vi "Run.vi"(8 "error in (no error)":errorcluster, 11 "S Parameter in":refnum<class "S Parameter.lvclass">) -> (0 "error out":errorcluster, 1 "Parameters":cluster{"Name":string, "Value":string}[](array[cluster]), 2 "Cancled":bool, 3 "S Parameter out":refnum<class "S Parameter.lvclass">)   [LabVIEW 2020, in "S Parameter.lvclass"]
doc: "This is the main test vi. It is here that the test is implemented."
uses:
  S Parameter.lvclass
  C:/Sandbox/Git_Sandbox/WiSpry Test Framework source code (LV20)/WiSpry Test Framework/Measurements/Measurement.lvclass
  Instruments/Vector Network Analyzer/Controls/Sparameter cluster.ctl
  Controls/Run States.ctl
  S Parameter.lvclass/S Parameter.ctl
  Instruments/Vector Network Analyzer/Vector Network Analyzer.lvclass/Vector Network Analyzer.ctl
  Instruments/Instrument.lvclass/Instrument.ctl
  Measurement.lvclass/Measurement.ctl
  XML Handler/XML Handler.lvclass/XML Handler.ctl
  Instruments/Power Supply/Power Supply.lvclass/Power Supply.ctl
  Devices/Controls/Change setting mode enum.ctl
  XML Handler/Controls/Result Cluster.ctl
  Instruments/Vector Network Analyzer/Vector Network Analyzer.lvclass
  C:/Sandbox/Git_Sandbox/WiSpry Test Framework source code (LV20)/WiSpry Test Framework/Instruments/Instrument.lvclass
  Support VI/Update parameters (array).vi
  Measurement.lvclass
  Devices/Device.lvclass
  Instruments/Power Supply/Power Supply.lvclass
  XML Handler/XML Handler.lvclass
  Devices/PIC-device/PIC-Device.lvclass
  Instruments/Digital Multimeter/Digital Multimeter.lvclass
  Instruments/Instrument.lvclass
  <vilib>/addons/HF Network Analysis/NI_HFNetworkAnalysis.lvlib
panel:
  out "S parameters":T1[](array[typedef])
  out "s-para plot error":errorcluster
  in  "S-par":u16(ring)
  in  "Format":u16(ring) items=["Ampl (dB)", "Ampl (mag)", "Phase (deg)", "Phase (rad)", "Re", "Im"]
  out "S-parameter Graph":T2(graph)
  out "Device Parameters":string
  out "Progress":u8(slide) scale=0.0..100.0
  in  "Cancel Button":bool
  out "Estimated finish time":timestamp format="%<%X>T"
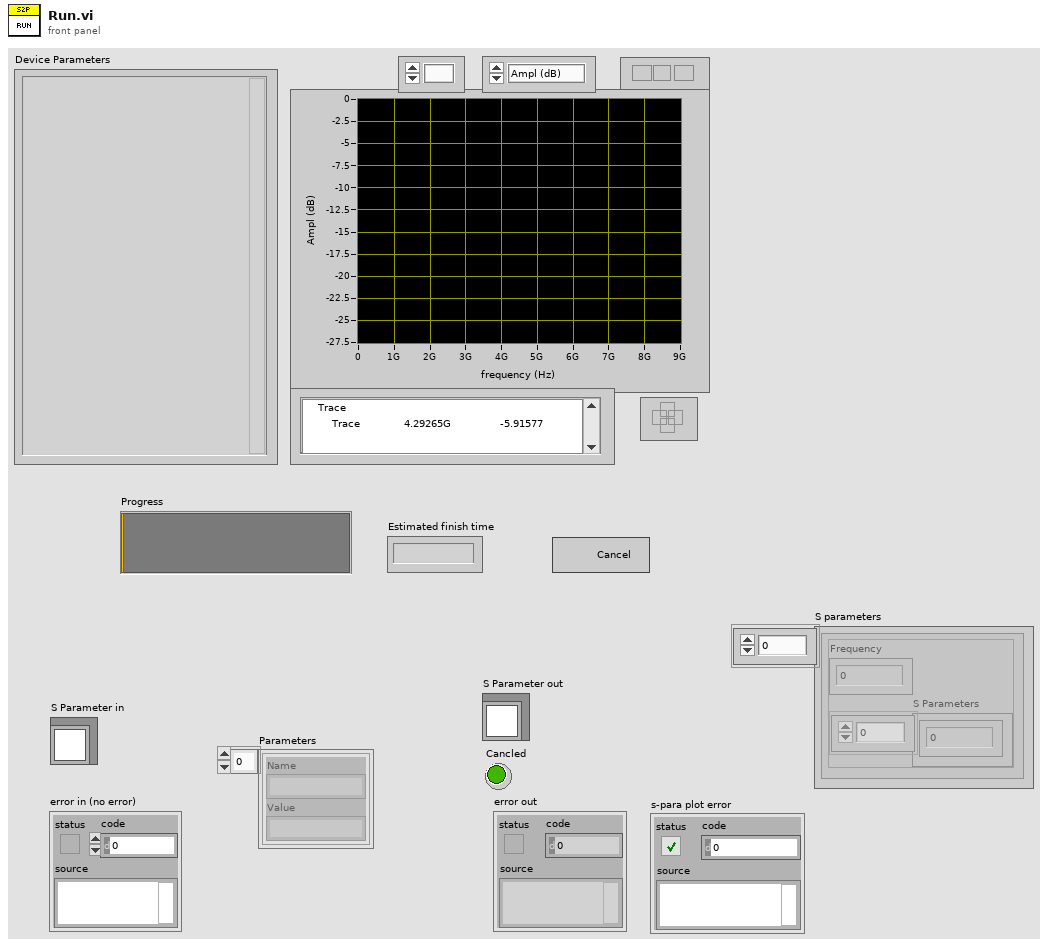
[diagram p1: front panel]
types:
  T1 = typedef "Vector Network Analyzer.lvclass/Sparameter cluster.ctl" = cluster{"Frequency":dbl, "S Parameters":cdb[]}
  T2 = cluster{"FrequencyList":dbl[], "Array out":dbl[]}
  T3 = typedef "Measurement.lvclass/Run States.ctl" = enum16{"Init", "Set Device", "Read Environment", "Measure", "Done"}
  T4 = typedef "PIC-Device.lvclass/Change setting mode enum.ctl" = enum16{"Init", "Next", "Reset"}
  T5 = typedef "XML Handler.lvclass/Result Cluster.ctl" = cluster{"Name":string, "Value":string}
  T6 = typedef "Device.lvclass/Device Information Cluster.ctl" = cluster{"Device Info":string[][], "Default Values":T7[], "Fetched info":string[][]}
  T7 = typedef "PIC-Device.lvclass/Register to Write.ctl" = cluster{"Register":u32, "Value":u32, "Dev Address":u32, "Physical Adress":u32}
  T8 = typedef "Instrument.lvclass/Interface String Cluster.ctl" = cluster{"Interface":string, "IDN string":string, "Instance":i32}
  T9 = cluster{"enabled":bool, "De-embed":bool, "Swap Ports Left":bool, "De-embedding file":path}[]
  T10 = cluster{"Frequencies":dbl[], "Formatted S-parameter":dbl[]}
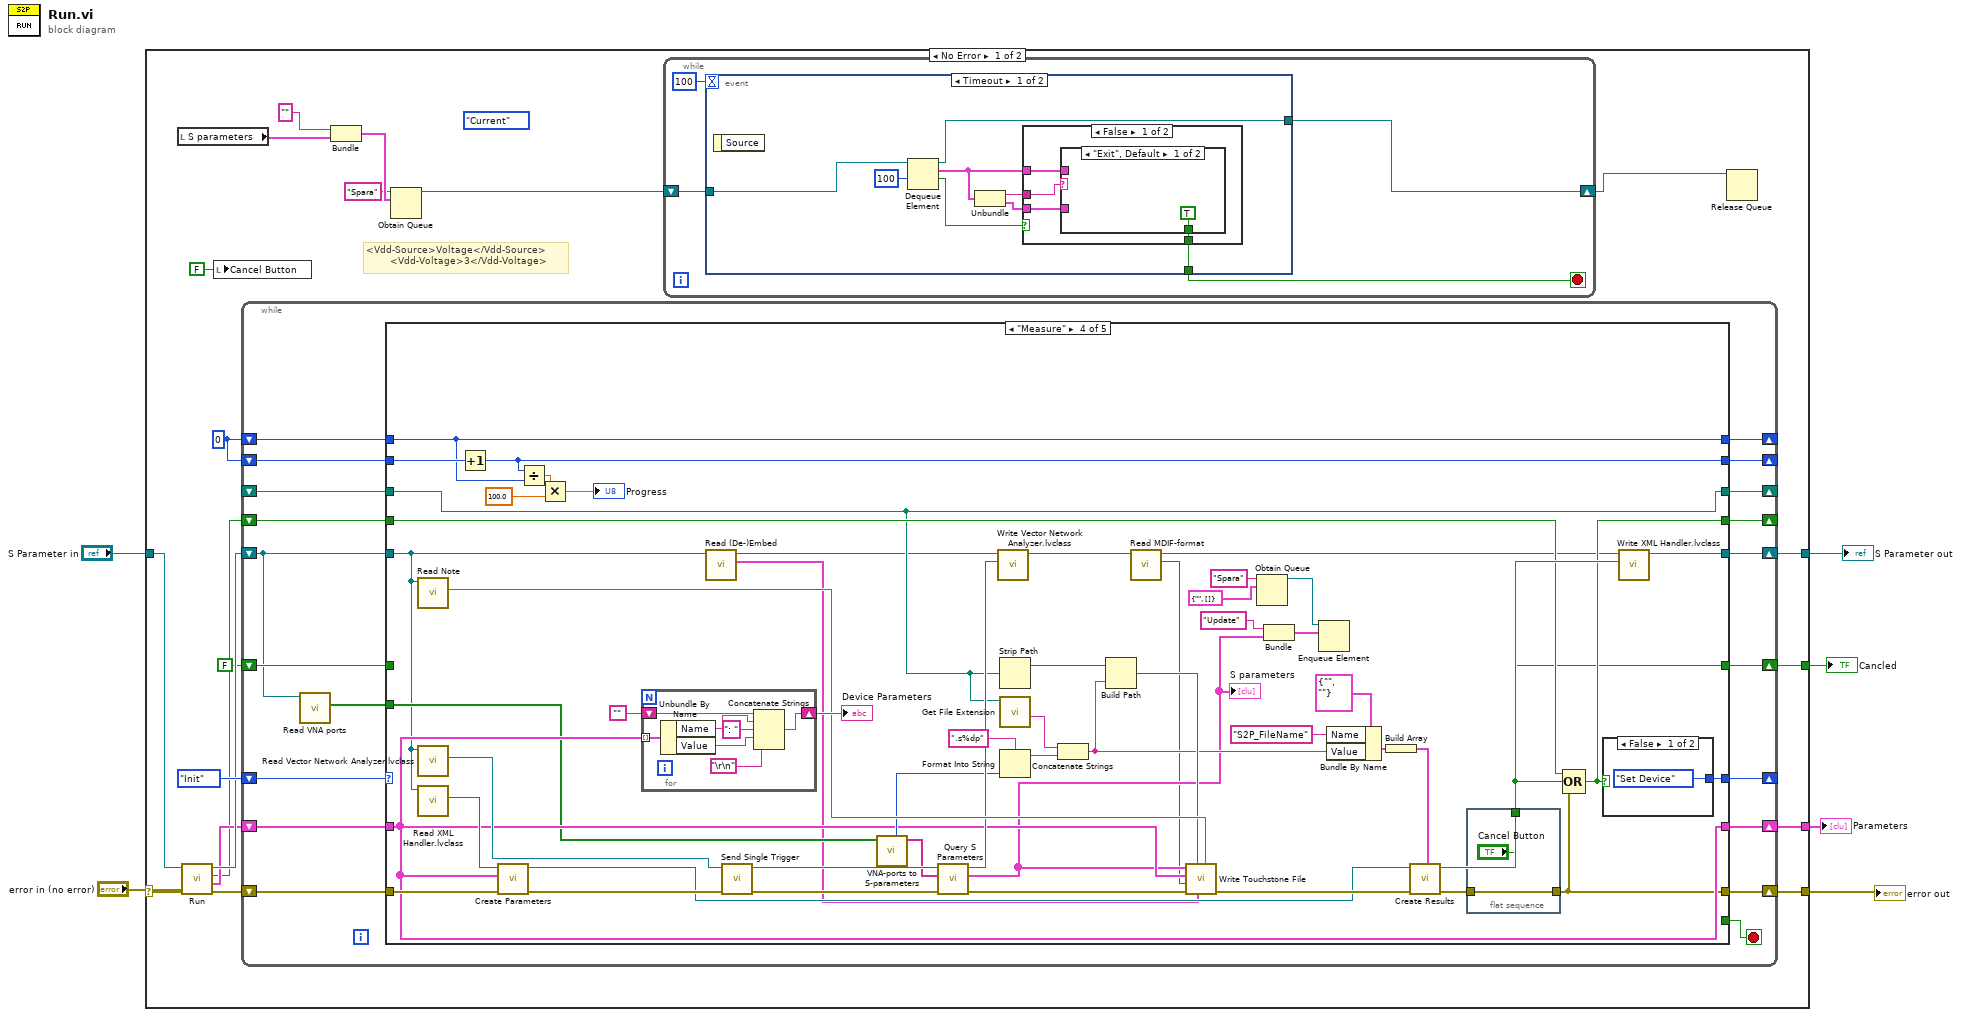
[diagram p0: block diagram]
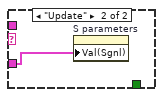
[diagram p2: hidden frame]
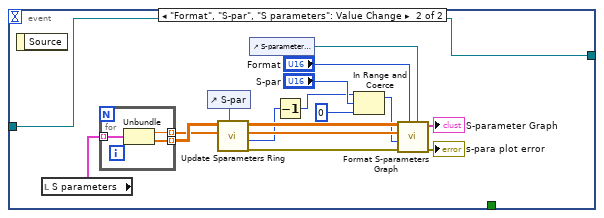
[diagram p4: hidden frame]
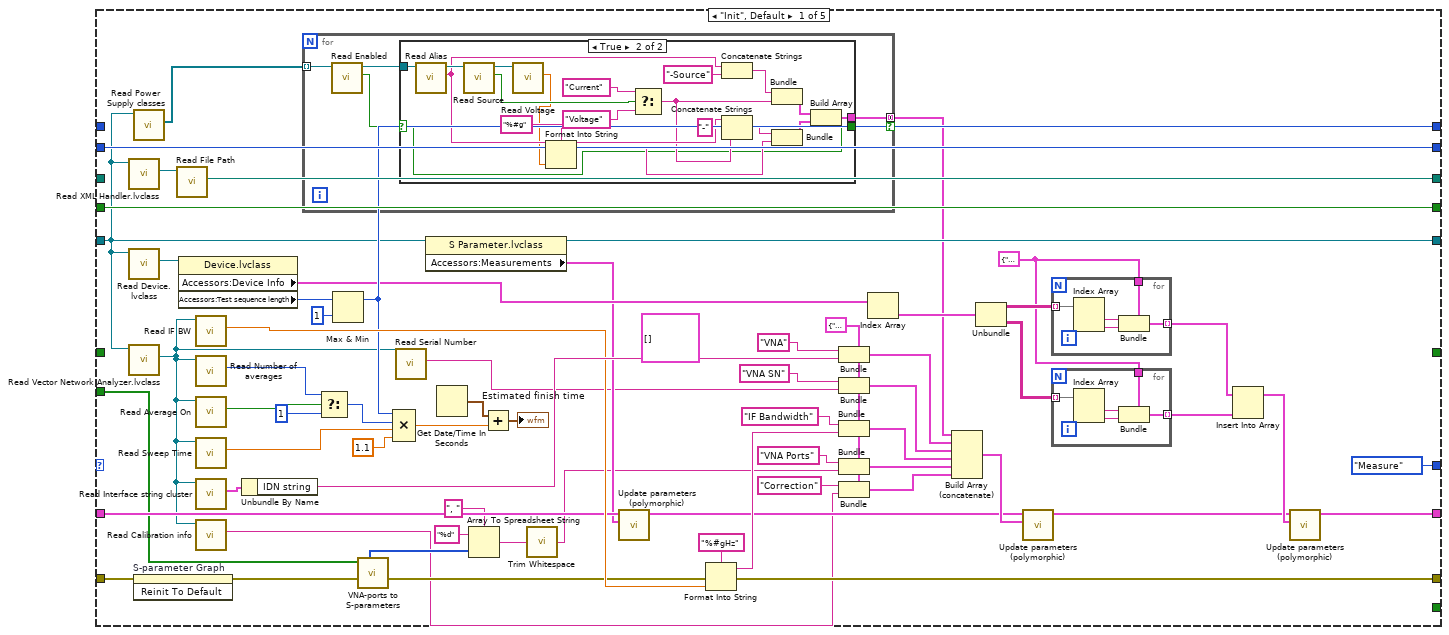
[diagram p5: hidden frame]
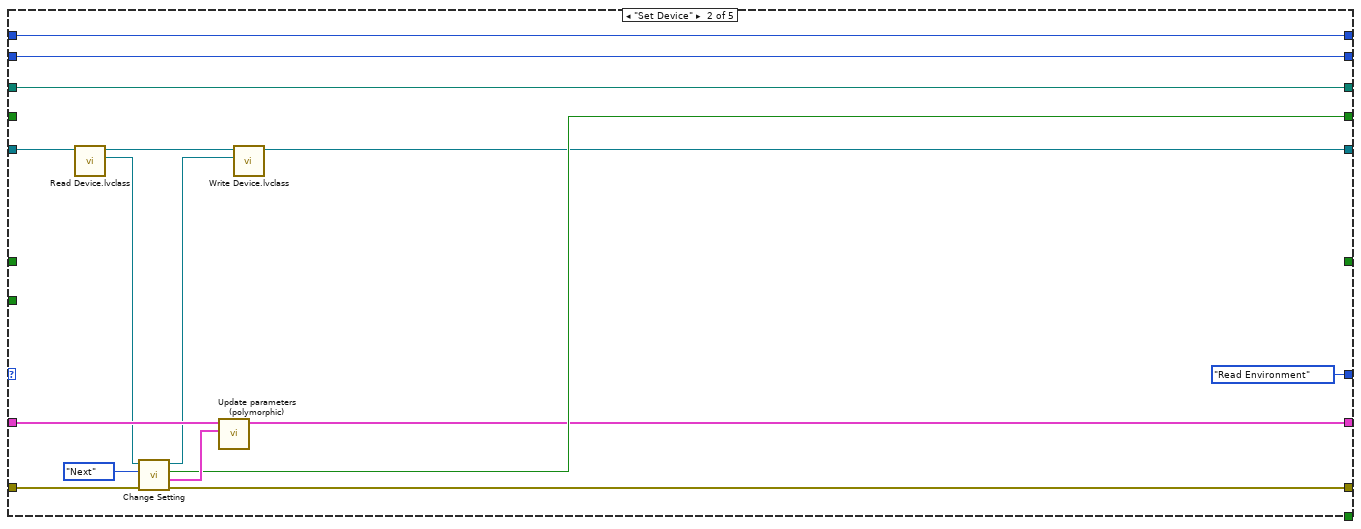
[diagram p7: hidden frame]
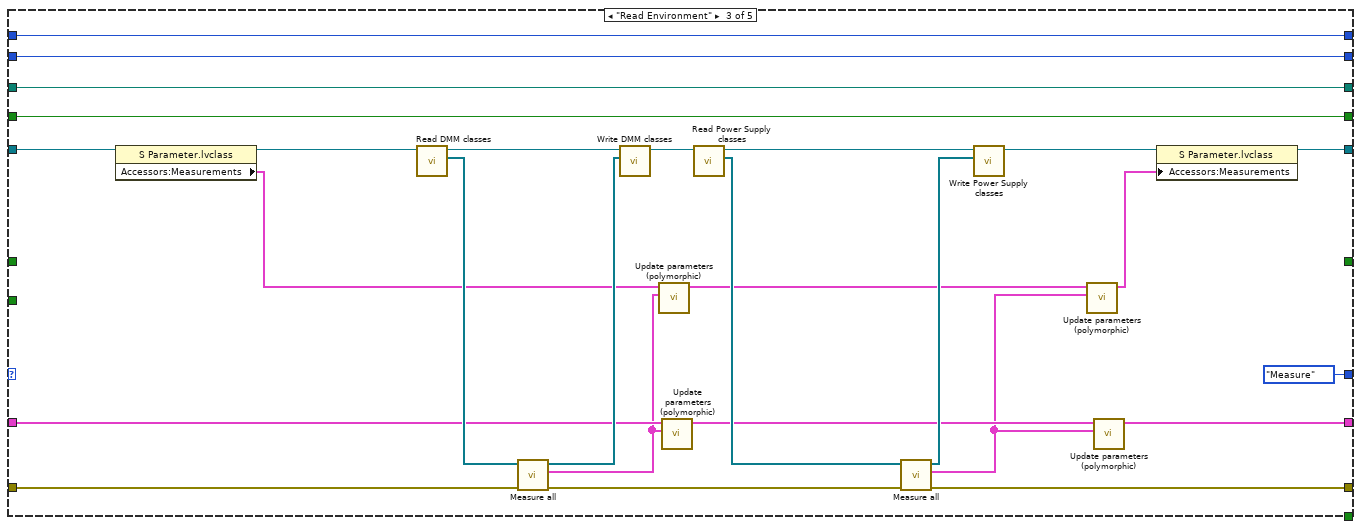
[diagram p8: hidden frame]
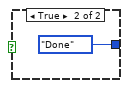
[diagram p9: hidden frame]
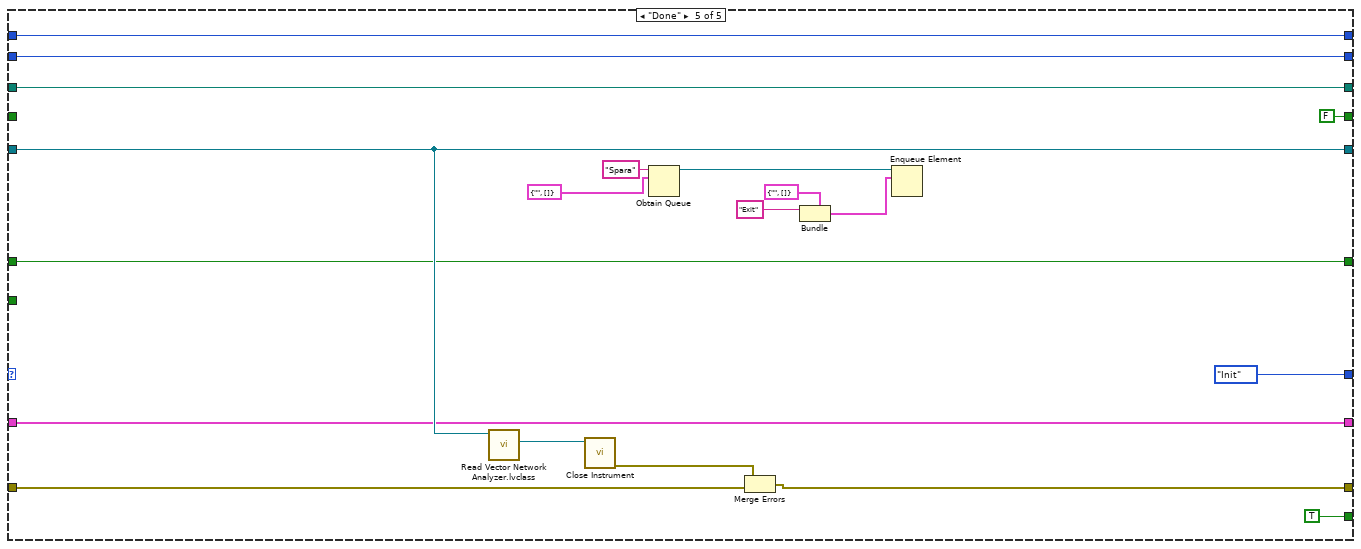
[diagram p10: hidden frame]
diagram:
  n1 = case shown="No Error" "error in (no error)" {
    selector: "error in (no error)" -> [w21 w311]
    tunnel: "S Parameter in" -> [w19 w312]
    tunnel: [w24 _] -> w4
    tunnel: [w23 w311] -> w3
    tunnel: [w22 w312] -> w2
    tunnel: [w17 _] -> w1
    frame No Error {
      (unwired) enum32{"Voltage", "Current"}."Current" ("Source")
      w25 = 0
      # "<Vdd-Source>Voltage</Vdd-Source>\n        <Vdd-Voltage>3</Vdd-Voltage>"
      n2 = local read "S parameters"() -> (w12:T1[])
      n3 = call-parent "Run.vi"("error in (no error)"=w21, "Measurements in"=w19) -> ("error out"=w20:errorcluster, "Parameters"=w16:cluster{"Name":string, "Value":string}[], "Canceled"=w15:bool, "Measurements out"=w18:refnum<class "S Parameter.lvclass">)  [unwired: 6 in]
      n4 = local write "Cancel Button"(FALSE ("Cancel Button")) -> ()
      n5 = while {
        shift-right: [w81] -> _
        shift-left: w25 -> [w83]
        shift-right: [w80] -> _
        shift-left: w25 -> [w82]
        shift-right: [w79] -> _
        shift-left: Run_States."Init" -> [w84]
        shift-right: [w77] -> w23
        shift-left: w20 -> [w78]
        shift-right: [w76] -> _
        shift-left: _ -> [w75]
        shift-right: [w74] -> w22
        shift-left: w18 -> [w66]
        shift-right: [w71] -> w17
        shift-left: w16 -> [w72]
        shift-right: [w70] -> _
        shift-left: w15 -> [w69]
        shift-right: [w65] -> w24
        shift-left: FALSE ("Cancel Button") -> [w67]
        stop <- w73 stop-if-true
        n6 = call-dynamic "Read VNA ports.vi"("S Parameter in"=w66) -> ("VNA ports"=w68:bool[])  [unwired: 9 in, 1 out]
        n7 = case shown="\"Measure\"" w84 {
          tunnel: w66 -> [w91 w190 w210 w228 w308]
          tunnel: w83 -> [_ w199 w226 w279 w310]
          tunnel: w82 -> [w146 w198 w225 w280 w303]
          tunnel: [w117 w199 w226 w279 w310] -> w81
          tunnel: [w146 w198 w225 w256 w303] -> w80
          tunnel: [Run_States."Measure" Run_States."Read Environment" Run_States."Measure" w258 Run_States."Init"] -> w79
          tunnel: w78 -> [w101 w192 w213 w248 w307]
          tunnel: [w124 w193 w217 w235 w304] -> w77
          tunnel: [w135 w197 w224 w244 w309] -> w76
          tunnel: w75 -> [_ w197 w224 w244 w309]
          tunnel: [w112 w185 w206 w272 w308] -> w74
          tunnel: [_ _ _ w233 w295] -> w65
          tunnel: [_ _ _ _ TRUE] -> w73
          tunnel: w72 -> [w110 w191 w202 w247 w301]
          tunnel: [w118 w187 w204 w247 w301] -> w71
          tunnel: [w136 w189 w222 w245 FALSE ("Last setting")] -> w70
          tunnel: w69 -> [w136 _ w222 w246 _]
          tunnel: w68 -> [w108 _ _ w239 _]
          tunnel: w67 -> [_ _ _ _ w295]
          frame "Init", Default {
            (unwired) cluster{"Name":string, "Value":string}[] [] ("Parameters Out")
            w94 = cluster{"Name":string, "Value":string} {"Name"="", "Value"=""} ("New Parameter")
            w96 = cluster{"Name":string, "Value":string} {"Name"="", "Value"=""} ("New Parameter")
            n8 = call "Read XML Handler.lvclass.vi"("Measurements in"=w91) -> ("XML Handler.lvclass"=w142:refnum<class "XML Handler.lvclass">)  [unwired: 9 in, 1 out]
            n9 = call "Read Device.lvclass.vi"("Measurements in"=w91) -> ("Device.lvclass"=w115:refnum<class "Device.lvclass">)  [unwired: 9 in, 1 out]
            n10 = call "Read Vector Network Analyzer.lvclass.vi"("S Parameter in"=w91) -> ("Vector Network Analyzer.lvclass"=w88:refnum<class "Vector Network Analyzer.lvclass">)  [unwired: 9 in, 1 out]
            n11 = call-dynamic "Read Power Supply classes.vi"("Measurements in"=w91) -> ("Power Supply classes"=w90:refnum<class "Power Supply.lvclass">[])  [unwired: 9 in, 1 out]
            n12 = invoke on="S-parameter Graph" class="XYGraph (strict)" method="Reinit To Default"(error in=w101) -> (error out=w100:errorcluster)  [unwired: 2 in, 2 out]
            n13 = call "Read File Path.vi"("XML Handler in"=w142) -> ("File Path"=w135:path)  [unwired: 9 in, 1 out]
            n14 = property class="Device.lvclass"(reference=w115) -> ("Accessors:Device Info"=w113:T6[], "Accessors:Test sequence length"=w114:i32)  [unwired: 1 in, 2 out]
            n15 = call "Read IF BW.vi"("Vector Network Analyzer in"=w88) -> ("IF BW"=w126:dbl)  [unwired: 9 in, 1 out]
            n16 = call "Read Number of averages.vi"("Vector Network Analyzer in"=w88) -> ("Number of averages"=w140:i32)  [unwired: 9 in, 1 out]
            n17 = call "Read Average On.vi"("Vector Network Analyzer in"=w88) -> ("Average On"=w141:bool)  [unwired: 9 in, 1 out]
            n18 = call "Read Sweep Time.vi"("Vector Network Analyzer in"=w88) -> ("Sweep Time"=w147:dbl)  [unwired: 9 in, 1 out]
            n19 = call "Read Interface string cluster.vi"("Instrument in"=w88) -> ("Interface sting cluster"=w132:T8)  [unwired: 9 in, 1 out]
            n20 = call-dynamic "Read Calibration info.vi"("Vector Network Analyzer in"=w88) -> ("Calibration info"=w97:string)  [unwired: 9 in, 1 out]
            n21 = Unbundle By Name(w132) -> ("IDN string"=w131:string)
            n22 = for {
              tunnel: w90 -> [w153] mode=indexing
              tunnel: [w150] -> w89 mode=concatenating if=w149
              n23 = call-dynamic "Read Enabled.vi"("Power Supply in"=w153) -> ("Enabled"=w152:bool, "Power Supply out"=w151:refnum<class "Power Supply.lvclass">)  [unwired: 9 in]
              n24 = case shown="True" w152 {
                selector: w152 -> [w154 w155]
                tunnel: w151 -> [_ w171]
                tunnel: [_ w156] -> w150
                tunnel: [w154 w155] -> w149
                frame False {
                }
                frame True {
                  n25 = call-dynamic "Read Alias.vi"("Power Supply in"=w171) -> ("Alias"=w163:string, "Power Supply out"=w173:refnum<class "Power Supply.lvclass">)  [unwired: 9 in]
                  n26 = call-dynamic "Read Source.vi"("Power Supply in"=w173) -> ("Source"=w168:bool, "Power Supply out"=w172:refnum<class "Power Supply.lvclass">)  [unwired: 9 in]
                  n27 = call "Read Voltage.vi"("Power Supply in"=w172) -> ("Voltage"=w160:dbl)  [unwired: 9 in, 1 out]
                  n28 = Format Into String(format string="%#g", w160) -> (resulting string=w159:string)  [unwired: 2 in, 1 out]
                  n29 = Select(t="Current" ("name (unnamed)"), s=w168, f="Voltage" ("name (unnamed)")) -> (s? t:f=w162:string)
                  n30 = Concatenate Strings(w163, "-Source" ("string")) -> (w167:string)
                  n31 = Concatenate Strings(w163, "-" ("string"), w162) -> (w164:string)
                  n32 = Bundle(w167, "name (unnamed)"=w162) -> (w158:cluster{string, "name (unnamed)":string})  [unwired: 1 in]
                  n33 = Bundle(w164, w159) -> (w157:cluster{string, string})  [unwired: 1 in]
                  n34 = Build Array(w158, w157) -> (w156:cluster{string, "name (unnamed)":string}[])
                }
              }
            }
            n35 = Select(t=w140, s=w141, f=1) -> (s? t:f=w138:i32)
            n36 = Max & Min(x=w114, y=1) -> (max(x,y)=w117:i32)  [unwired: 1 out]
            n37 = call "VNA-ports to S-parameters.vi"("VNA ports"=w108) -> ("Port numbers"=w107:i32[])  [unwired: 6 in, 4 out]
            n38 = Compound Arithmetic op=MULTIPLY(w117, w138, w147, 1.1 ("value")) -> (w145:dbl)
            n39 = call-dynamic "Read Serial Number.vi"("Instrument in"=w88) -> ("Serial Number"=w86:string)  [unwired: 9 in, 1 out]
            n40 = property class="S Parameter.lvclass"(reference=w91) -> (reference out=w112:refnum<class "S Parameter.lvclass">, "Accessors:Measurements"=w109:cluster{"Name":string, "Value":string}[])  [unwired: 1 in, 1 out]
            n41 = Get Date/Time In Seconds() -> (seconds since 1Jan1904=w143:timestamp)
            n42 = Array To Spreadsheet String(delimiter (Tab)=", ", array=w107, 3:"%d" ("format string")) -> (spreadsheet string=w103:string)
            n43 = Add(x=w143, y=w145) -> (x+y=→"Estimated finish time":timestamp)
            n44 = call <vilib>:"Trim Whitespace.vi"("string"=w103) -> ("trimmed string"=w102:string)  [unwired: 1 in]
            n45 = call-poly "Update parameters (polymorphic).vi"("New Parameters"=w109, "Parameters"=w110) -> ("Parameters Out"=w111:cluster{"Name":string, "Value":string}[])  [unwired: 9 in]
            n46 = Format Into String(format string="%#gHz", error in=w100, w126) -> (resulting string=w125:string, error out=w124:errorcluster)  [unwired: 1 in]
            n47 = Bundle(cluster=w96, "Name"="VNA", "Value"=w131) -> (w130:cluster{"Name":string, "Value":string})
            n48 = Bundle("Name"="VNA SN", "Serial Number"=w86) -> (w85:cluster{"Name":string, "Serial Number":string})  [unwired: 1 in]
            n49 = Bundle(cluster=w96, "Name"="IF Bandwidth", "Value"=w125) -> (w129:cluster{"Name":string, "Value":string})
            n50 = Bundle(cluster=w96, "Name"="VNA Ports", "Value"=w102) -> (w98:cluster{"Name":string, "Value":string})
            n51 = Bundle(cluster=w96, "Name"="Correction", "Value"=w97) -> (w95:cluster{"Name":string, "Value":string})
            n52 = Index Array(array=w113) -> (element=w123:T6)  [unwired: 1 in]
            n53 = Build Array (concatenate)(w89, w130, w85, w129, w98, w95) -> (w128:cluster{"Name":string, "Value":string}[])
            n54 = Unbundle(w123) -> ("Device Info"=w121:string[][], "Fetched info"=w93:string[][])  [unwired: 1 out]
            n55 = call-poly "Update parameters (polymorphic).vi"("New Parameters"=w128, "Parameters"=w111) -> ("Parameters Out"=w119:cluster{"Name":string, "Value":string}[])  [unwired: 9 in]
            n56 = for {
              tunnel: w94 -> [w183]
              tunnel: [w179] -> w122 mode=indexing
              tunnel: w121 -> [w182] mode=indexing
              n57 = Index Array(array=w182) -> (element #1=w181:string, element #2=w180:string)  [unwired: 2 in]
              n58 = Bundle(cluster=w183, "Name"=w181, "Value"=w180) -> (w179:cluster{"Name":string, "Value":string})
            }
            n59 = for {
              tunnel: w94 -> [w178]
              tunnel: [w174] -> w92 mode=indexing
              tunnel: w93 -> [w177] mode=indexing
              n60 = Index Array(array=w177) -> (element #1=w176:string, element #2=w175:string)  [unwired: 2 in]
              n61 = Bundle(cluster=w178, "Name"=w176, "Value"=w175) -> (w174:cluster{"Name":string, "Value":string})
            }
            n62 = Insert Into Array(array=w122, new element=w92) -> (w120:cluster{"Name":string, "Value":string}[])  [unwired: 1 in]
            n63 = call-poly "Update parameters (polymorphic).vi"("New Parameters"=w120, "Parameters"=w119) -> ("Parameters Out"=w118:cluster{"Name":string, "Value":string}[])  [unwired: 9 in]
          }
          frame "Set Device" {
            n64 = call "Read Device.lvclass.vi"("Measurements in"=w190) -> ("Device.lvclass"=w188:refnum<class "Device.lvclass">, "Measurements out"=w186:refnum<class "S Parameter.lvclass">)  [unwired: 9 in]
            n65 = call-dynamic "Change Setting.vi"("error in (no error)"=w192, "Change setting mode"=Change_setting_mode_enum."Next", "Device in"=w188) -> ("error out"=w193:errorcluster, "Changes"=w194:cluster{"Name":string, "Value":string}[], "Last setting"=w189:bool, "Device out"=w184:refnum<class "Device.lvclass">)  [unwired: 5 in]
            n66 = call-poly "Update parameters (polymorphic).vi"("New Parameters"=w194, "Parameters"=w191) -> ("Parameters Out"=w187:cluster{"Name":string, "Value":string}[])  [unwired: 9 in]
            n67 = call "Write Device.lvclass.vi"("Device.lvclass"=w184, "Measurements in"=w186) -> ("Measurements out"=w185:refnum<class "S Parameter.lvclass">)  [unwired: 9 in]
          }
          frame "Read Environment" {
            n68 = property class="S Parameter.lvclass"(reference=w210) -> (reference out=w209:refnum<class "S Parameter.lvclass">, "Accessors:Measurements"=w208:cluster{"Name":string, "Value":string}[])  [unwired: 1 in, 1 out]
            n69 = call-dynamic "Read DMM classes.vi"("Measurements in"=w209) -> ("DMM classes"=w215:refnum<class "Digital Multimeter.lvclass">[], "Measurements out"=w221:refnum<class "S Parameter.lvclass">)  [unwired: 9 in]
            n70 = call "Measure all.vi"("error in (no error)"=w213, "Digital Multimeters in"=w215) -> ("error out"=w212:errorcluster, "Measurements"=w201:T5[], "Digital Multimeters out"=w214:refnum<class "Digital Multimeter.lvclass">[])  [unwired: 5 in, 2 out]
            n71 = call-dynamic "Write DMM classes.vi"("DMM classes"=w214, "Measurements in"=w221) -> ("Measurements out"=w216:refnum<class "S Parameter.lvclass">)  [unwired: 9 in]
            n72 = call-poly "Update parameters (polymorphic).vi"("New Parameters"=w201, "Parameters"=w208) -> ("Parameters Out"=w211:cluster{"Name":string, "Value":string}[])  [unwired: 9 in]
            n73 = call-poly "Update parameters (polymorphic).vi"("New Parameters"=w201, "Parameters"=w202) -> ("Parameters Out"=w203:cluster{"Name":string, "Value":string}[])  [unwired: 9 in]
            n74 = call-dynamic "Read Power Supply classes.vi"("Measurements in"=w216) -> ("Power Supply classes"=w219:refnum<class "Power Supply.lvclass">[], "Measurements out"=w220:refnum<class "S Parameter.lvclass">)  [unwired: 9 in]
            n75 = call "Measure all.vi"("error in (no error)"=w212, "Power Supplies in"=w219) -> ("error out"=w217:errorcluster, "Measurements"=w200:T5[], "Power Supplies out"=w218:refnum<class "Power Supply.lvclass">[])  [unwired: 5 in, 2 out]
            n76 = call-dynamic "Write Power Supply classes.vi"("Power Supply classes"=w218, "Measurements in"=w220) -> ("Measurements out"=w207:refnum<class "S Parameter.lvclass">)  [unwired: 9 in]
            n77 = call-poly "Update parameters (polymorphic).vi"("New Parameters"=w200, "Parameters"=w211) -> ("Parameters Out"=w205:cluster{"Name":string, "Value":string}[])  [unwired: 9 in]
            n78 = call-poly "Update parameters (polymorphic).vi"("New Parameters"=w200, "Parameters"=w203) -> ("Parameters Out"=w204:cluster{"Name":string, "Value":string}[])  [unwired: 9 in]
            n79 = property class="S Parameter.lvclass"(reference=w207, "Accessors:Measurements"=w205) -> (reference out=w206:refnum<class "S Parameter.lvclass">)  [unwired: 1 in, 1 out]
          }
          frame "Measure" {
            n80 = call "Read Note.vi"("S Parameter in"=w228) -> ("Note"=w266:string)  [unwired: 9 in, 1 out]
            n81 = call "Read Vector Network Analyzer.lvclass.vi"("S Parameter in"=w228) -> ("Vector Network Analyzer.lvclass"=w270:refnum<class "Vector Network Analyzer.lvclass">)  [unwired: 9 in, 1 out]
            n82 = call "Read XML Handler.lvclass.vi"("Measurements in"=w228) -> ("XML Handler.lvclass"=w257:refnum<class "XML Handler.lvclass">)  [unwired: 9 in, 1 out]
            n83 = Increment(x=w280) -> (x+1=w256:i32)
            n84 = call "Create Parameters.vi"("error in (no error)"=w248, "Parameters"=w247, "XML Handler in"=w257) -> ("error out"=w271:errorcluster, "XML Handler out"=w261:refnum<class "XML Handler.lvclass">)  [unwired: 7 in]
            n85 = Divide(x=w256, y=w279) -> (x/y=w277:dbl)
            n86 = Multiply(x=w277, y=100.0) -> (x*y=→"Progress":dbl)
            n87 = for {
              tunnel: w247 -> [w291] mode=indexing
              shift-right: [w285] -> w274
              shift-left: "" -> [w290]
              n88 = Unbundle By Name(w291) -> ("Name"=w289:string, "Value"=w287:string)
              n89 = Concatenate Strings(w290, w289, ": " ("string"), w287, "\r\n") -> (w285:string)
            }
            "Device Parameters" <- w274
            n90 = call-dynamic "Read (De-)Embed.vi"("S Parameter in"=w228) -> ("(De-)Embed"=w229:T9, "S Parameter out"=w227:refnum<class "S Parameter.lvclass">)  [unwired: 9 in]
            n91 = call-dynamic "Send Single Trigger.vi"("error in (no error)"=w271, "Vector Network Analyzer in"=w270) -> ("error out"=w269:errorcluster, "Vector Network Analyzer out"=w268:refnum<class "Vector Network Analyzer.lvclass">)  [unwired: 8 in]
            n92 = call "VNA-ports to S-parameters.vi"("VNA ports"=w239) -> ("Sparameters (string)"=w254:string[], "Number of ports"=w251:i32)  [unwired: 6 in, 3 out]
            n93 = call-dynamic "Query S Parameters.vi"("error in (no error)"=w269, "Sparameters (string)"=w254, "Vector Network Analyzer in"=w268) -> ("error out"=w267:errorcluster, "S parameters"=w242:T1[], "Vector Network Analyzer out"=w253:refnum<class "Vector Network Analyzer.lvclass">)  [unwired: 6 in]
            "S parameters" <- w242
            n94 = call "Write Vector Network Analyzer.lvclass.vi"("Vector Network Analyzer.lvclass"=w253, "S Parameter in"=w227) -> ("S Parameter out"=w238:refnum<class "S Parameter.lvclass">)  [unwired: 9 in]
            n95 = Strip Path(path=w244) -> (stripped path=w249:path)  [unwired: 1 out]
            n96 = call <vilib>:"Get File Extension.vi"("file"=w244) -> ("filename without extension"=w243:string)  [unwired: 6 in, 4 out]
            n97 = Format Into String(format string=".s%dp" ("string"), w251) -> (resulting string=w250:string)  [unwired: 2 in, 1 out]
            n98 = Concatenate Strings(w243, w250) -> (w255:string)
            n99 = Build Path(base path=w249, name or relative path=w255) -> (appended path=w263:path)
            n100 = call-dynamic "Read MDIF-format.vi"("S Parameter in"=w238) -> ("MDIF-format"=w236:bool, "S Parameter out"=w237:refnum<class "S Parameter.lvclass">)  [unwired: 9 in]
            n101 = call "Write Touchstone File.vi"("Note"=w266, "(De-)Embed"=w229, "File Path"=w263, "Error In"=w267, "MDIF-format"=w236, "Parameters"=w247, "Sparameters"=w242) -> ("Error Out"=w262:errorcluster)  [unwired: 4 in]
            n102 = Obtain Queue(name (unnamed)="Spara", element data type=cluster{string, "S parameters":T1[]} {"", "S parameters"=[]} ("output cluster")) -> (queue out=w230:refnum<queue>)  [unwired: 3 in, 2 out]
            n103 = Bundle("Update", "S parameters"=w242) -> (w241:cluster{string, "S parameters":T1[]})  [unwired: 1 in]
            n104 = Enqueue Element(queue=w230, element=w241) -> ()  [unwired: 2 in, 3 out]
            n105 = Bundle By Name(cluster=T5 {"Name"="", "Value"=""} ("Result Cluster"), "Name"="S2P_FileName", "Value"=w255) -> (w260:T5)
            n106 = Build Array(w260) -> (w259:T5[])
            n107 = call "Create Results.vi"("error in (no error)"=w262, "Results"=w259, "XML Handler in"=w261) -> ("error out"=w234:errorcluster, "XML Handler out"=w273:refnum<class "XML Handler.lvclass">)  [unwired: 7 in]
            n108 = flat-sequence {
              tunnel: [w282] -> w235
              tunnel: w234 -> [w282]
              tunnel: ["Cancel Button"] -> w233
              frame #0 {
              }
            }
            n109 = Compound Arithmetic op=OR(w246, w233, w235) -> (w245:bool)
            n110 = case shown="False" w245 {
              tunnel: [Run_States."Set Device" Run_States."Done"] -> w258
              frame False {
              }
              frame True {
              }
            }
            n111 = call "Write XML Handler.lvclass.vi"("XML Handler.lvclass"=w273, "Measurements in"=w237) -> ("Measurements out"=w272:refnum<class "S Parameter.lvclass">)  [unwired: 9 in]
          }
          frame "Done" {
            n112 = call "Read Vector Network Analyzer.lvclass.vi"("S Parameter in"=w308) -> ("Vector Network Analyzer.lvclass"=w306:refnum<class "Vector Network Analyzer.lvclass">)  [unwired: 9 in, 1 out]
            n113 = call-dynamic "Close Instrument.vi"("Instrument in"=w306) -> ("error out"=w305:errorcluster)  [unwired: 9 in, 1 out]
            n114 = Obtain Queue(name (unnamed)="Spara", element data type=cluster{string, "S parameters":T1[]} {"", "S parameters"=[]} ("output cluster")) -> (queue out=w293:refnum<queue>)  [unwired: 3 in, 2 out]
            n115 = Merge Errors(w305, w307) -> (w304:errorcluster)
            n116 = Bundle(cluster=cluster{string, "S parameters":T1[]} {"", "S parameters"=[]}, "Exit") -> (w297:cluster{string, "S parameters":T1[]})  [unwired: 1 in]
            n117 = Enqueue Element(queue=w293, element=w297) -> ()  [unwired: 2 in, 3 out]
          }
        }
      }
      n118 = Bundle("", "S parameters"=w12) -> (w10:cluster{string, "S parameters":T1[]})  [unwired: 1 in]
      n119 = Obtain Queue(name (unnamed)="Spara", element data type=w10) -> (queue out=w14:refnum<queue>)  [unwired: 3 in, 2 out]
      n120 = while {
        shift-right: [w28] -> w13
        shift-left: w14 -> [w29]
        stop <- w27 stop-if-true
        n121 = event shown="[0] Timeout" {
          selector: _ -> [_ _]
          dyn-events: _ -> [_ _]
          timeout: 100 -> [_ _]
          tunnel: w29 -> [w37 w50]
          tunnel: [w35 w50] -> w28
          tunnel: [w31 _] -> w27
          event Timeout {
            n122 = event-data() -> ()  [unwired: 1 in, 1 out]
            n123 = Dequeue Element(queue=w37, timeout in ms (-1)=100) -> (queue out=w35:refnum<queue>, element=w34:cluster{string, "S parameters":T1[]}, timed out?=w36:bool)  [unwired: 1 in, 1 out]
            n124 = Unbundle(w34) -> (w33:string, "S parameters"=w32:T1[])
            n125 = case shown="False" w36 {
              tunnel: w34 -> [w42 _]
              tunnel: w33 -> [w41 _]
              tunnel: w32 -> [w40 _]
              tunnel: [w39 _] -> w31
              frame False {
                n126 = case shown="\"Exit\", Default" w41 {
                  tunnel: w42 -> [_ _]
                  tunnel: w40 -> [_ w44]
                  tunnel: [TRUE _] -> w39
                  frame "Exit", Default {
                  }
                  frame "Update" {
                    n127 = property on="S parameters" class="Arr (strict)"("Val(Sgnl)"=w44) -> ()  [unwired: 2 in, 2 out]
                  }
                }
              }
              frame True {
              }
            }
          }
          event "Format", "S-par", "S parameters": Value Change {
            n128 = event-data() -> ()  [unwired: 1 in, 1 out]
            n129 = local read "S parameters"() -> (w51:T1[])
            n130 = for {
              tunnel: w51 -> [w64] mode=indexing
              tunnel: [w63] -> w60 mode=indexing
              tunnel: [w62] -> w61 mode=indexing
              n131 = Unbundle(w64) -> ("Frequency"=w63:dbl, "S Parameters"=w62:cdb[])
            }
            n132 = control-ref of="S-par"() -> (w58:refnum<vi>)
            n133 = call <vilib>:"Update Sparameters Ring.vi"("S-par reference"=w58, "Frequencies in"=w60, "S-parameters in"=w61) -> ("error out"=w54:errorcluster, "Number of S-parameters"=w47:i32, "Frequencies out"=w56:dbl[], "S-parameters out"=w55:cdb[][])  [unwired: 5 in]
            n134 = control-ref of="S-parameter Graph"() -> (w53:refnum<vi>)
            n135 = Decrement(x=w47) -> (x-1=w46:i32)
            n136 = In Range and Coerce(upper limit=w46, x="S-par", lower limit=0) -> (coerced(x)=w48:i32)  [unwired: 1 out]
            n137 = call <vilib>:"Format S-parameters Graph.vi"("S-parameter reference"=w53, "Format"="Format", "error in (no error)"=w54, "S-parameter Index"=w48, "Frequencies"=w56, "S-parameters"=w55) -> ("error out"=→"s-para plot error":errorcluster, "S-parameter Graph"=→"S-parameter Graph":T10)  [unwired: 4 in]
          }
        }
      }
      n138 = Release Queue(queue=w13) -> ()  [unwired: 2 in, 3 out]
    }
    frame Error {
    }
  }
  "error out" <- w3
  "S Parameter out" <- w2
  "Cancled" <- w4
  "Parameters" <- w1
